vi "new.vi"(8 "error in (no error)":errorcluster, 11 "interface in":refnum<class "interface.lvclass">) -> (0 "error out":errorcluster, 3 "interface out":refnum<class "interface.lvclass">)   [LabVIEW 2015, in "example_01.lvlib" / "functional.lvlib" / "interface.lvclass"]
uses:
  interface.lvclass
  _controls/event_data.ctl
  _controls/event_command.ctl
  interface.lvclass/interface.ctl
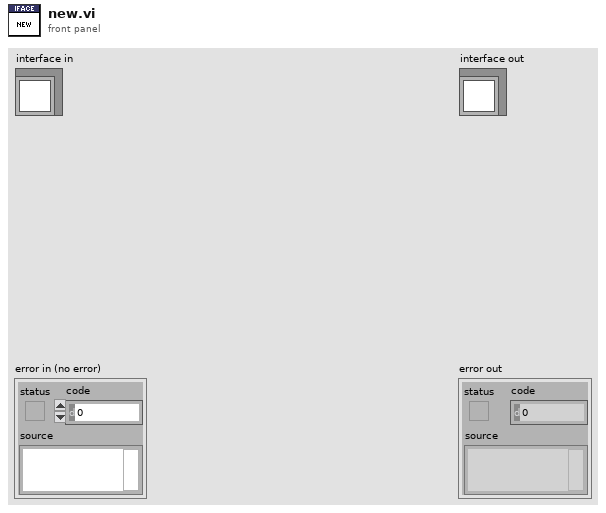
[diagram p1: front panel]
types:
  T1 = typedef "example_01.lvlib/functional.lvlib/interface.lvclass/event_data.ctl" = cluster{"command":T2, "data":variant}
  T2 = typedef "example_01.lvlib/functional.lvlib/interface.lvclass/event_command.ctl" = enum16{"<event_command>", "stop", "<null>"}
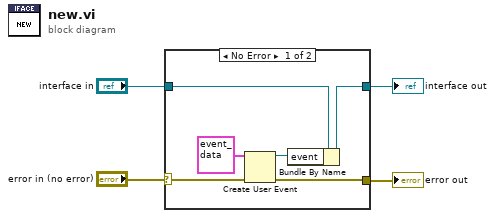
[diagram p0: block diagram]
diagram:
  n1 = case shown="No Error" "error in (no error)" {
    selector: "error in (no error)" -> [w7 w12]
    tunnel: [w5 w12] -> w3
    tunnel: "interface in" -> [w10 w11]
    tunnel: [w9 w11] -> w1
    frame No Error {
      n2 = Create User Event(user event datatype=T1 {"command"=enum."<event_command>", "data"=variant} ("event"), error in=w7) -> (user event=w6:refnum<user-event>, error out=w5:errorcluster)
      n3 = Bundle By Name(cluster=w10, "event"=w6) -> (w9:refnum<class "interface.lvclass">)
    }
    frame Error {
    }
  }
  "error out" <- w3
  "interface out" <- w1
